vi "zad1.vi"() -> ()   [LabVIEW 2018]
uses:
  Control 6.ctl
  Control 1.ctl
  Control 3.ctl
  <vilib>/measure/maspectr.llb/FFT Power Spectrum and PSD for 1 Chan.vi
  <vilib>/measure/NI_MAPro.lvlib
panel:
  out "Waveform Graph 2":cluster{"f0":dbl, "df":dbl, "magnitude":dbl[]}(graph)
  in  "millisec to wait":u32
  in  "idev 2":u32
  in  "Buffer":T1
  in  "Format":cluster{"Rate":i32, "Bits":i32, "Channels":u32}
  in  "Play":bool
  in  "Exit":bool
  out "Waveform Graph":i32[][](graph)
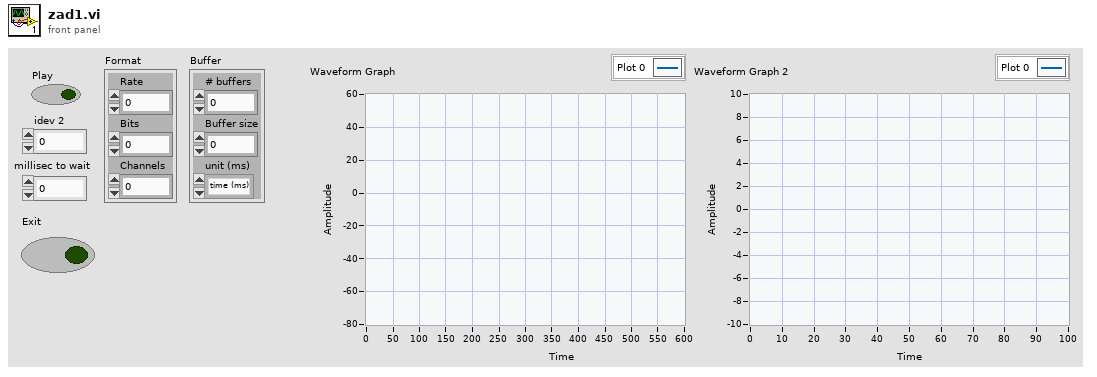
[diagram p1: front panel]
types:
  T1 = cluster{"# buffers":i32, "Buffer size":i32, "unit (ms)":enum16{"time (ms)", "Samples"}}
  T2 = typedef "Control 1.ctl" = enum16{"Analysis", "Initialization", "Idle"}
  T3 = typedef "Control 6.ctl" = enum16{"Idle", "Initialization", "Acquisition", "End"}
  T4 = typedef "Control 3.ctl" = cluster{"Play":bool, "Format (44kHz, 16Bit, stereo)":cluster{"Rate":i32, "Bits":i32, "Channels":u32}, "Buffer Config":cluster{"# buffers":i32, "Buffer size":i32, "unit (ms)":enum16{"time (ms)", "Samples"}}, "idev":u32, "millisec to wait":u32}
  T5 = enum16{"Idle", "Initialization", "Acquisition", "End"}
  T6 = typedef "Control 4.ctl" = cluster{"Play":bool, "Format (44kHz, 16Bit, stereo)":cluster{"Rate":i32, "Bits":i32, "Channels":u32}, "Buffer Config":cluster{"# buffers":i32, "Buffer size":i32, "unit (ms)":enum16{"time (ms)", "Samples"}}, "idev":u32, "millisec to wait":u32}
  T7 = typedef "SoundHandle.ctl" = cluster{"DeviceID":u16, "Samples/buf":u32, "Sampl rate":u32, "Bits/sample":u16, "Channels":u8, "Opened":bool}
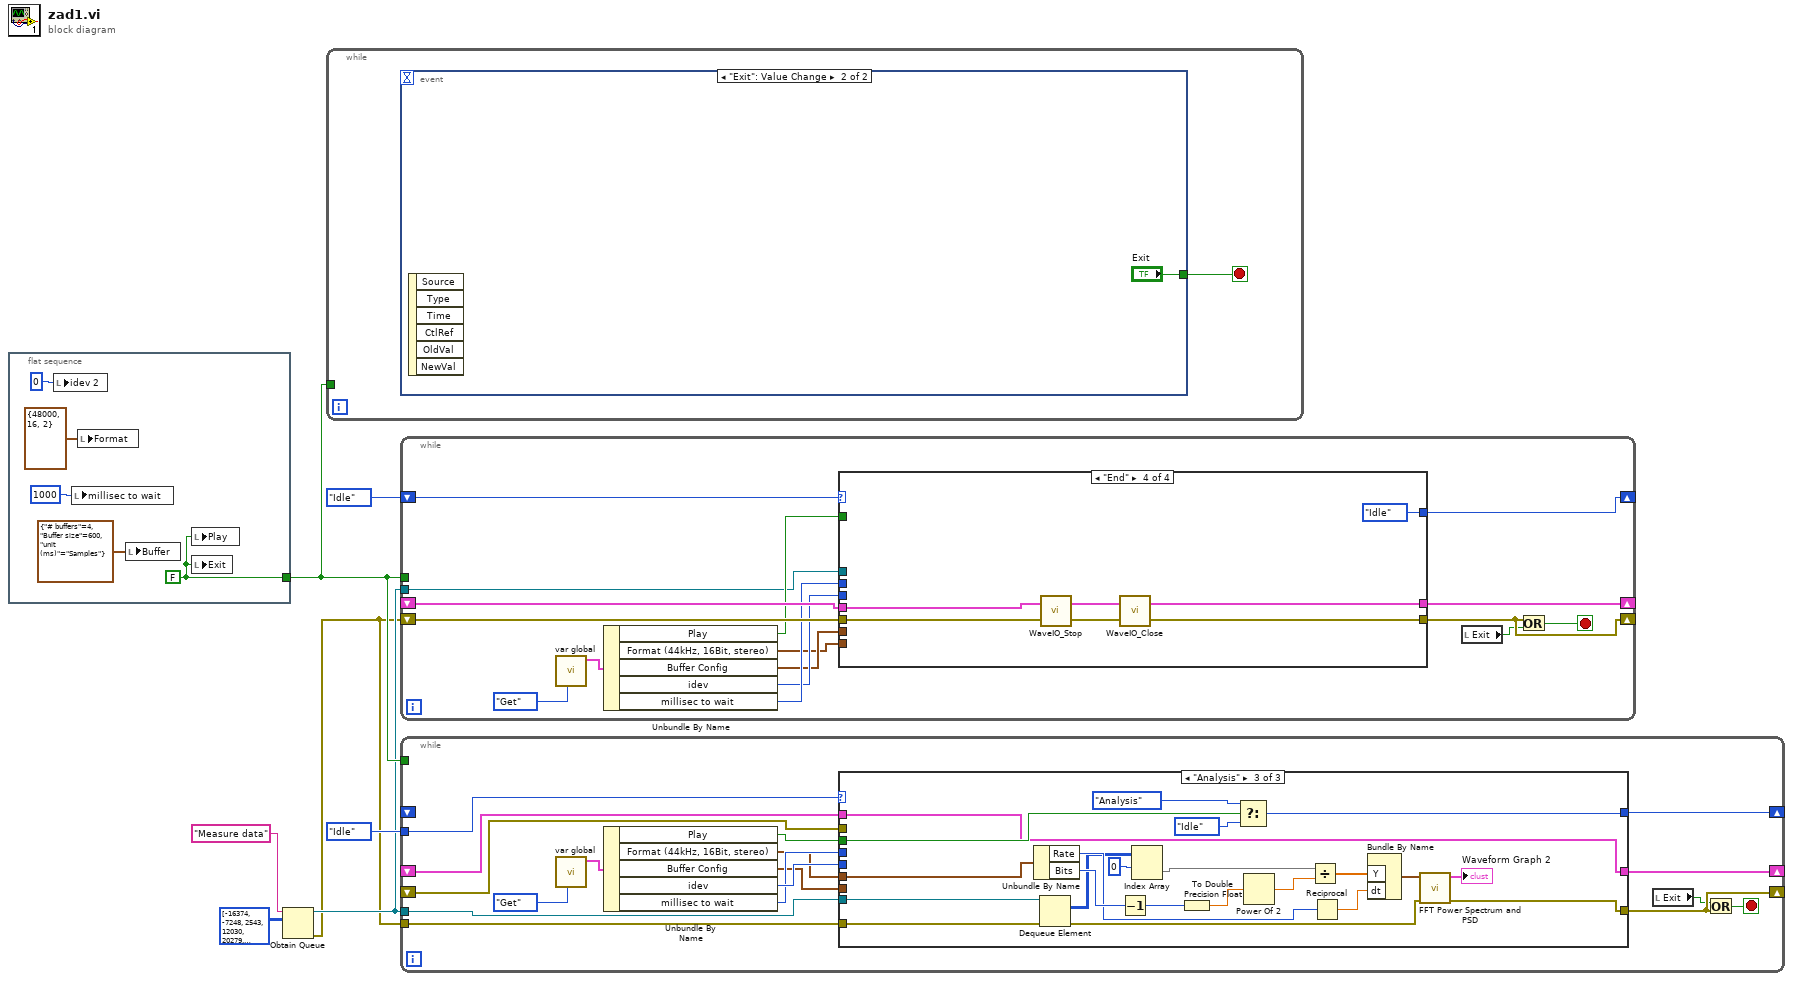
[diagram p0: block diagram]
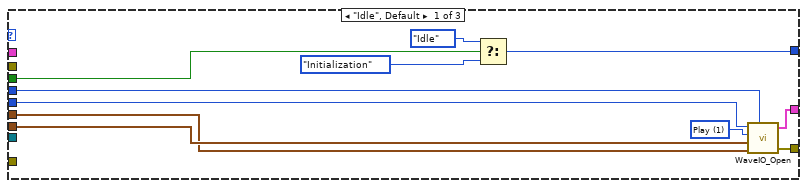
[diagram p2: hidden frame]
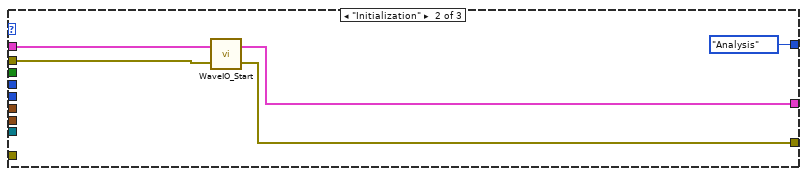
[diagram p3: hidden frame]
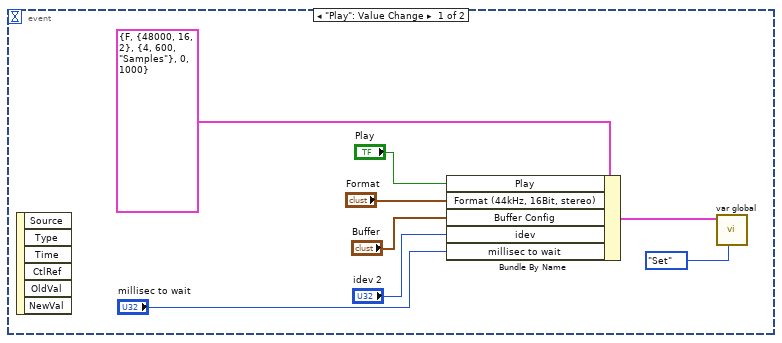
[diagram p4: hidden frame]
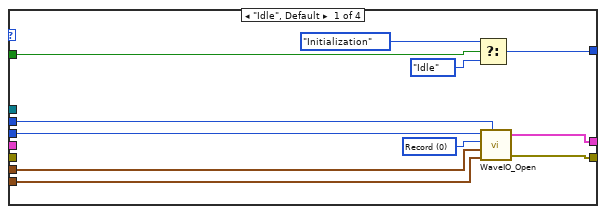
[diagram p5: hidden frame]
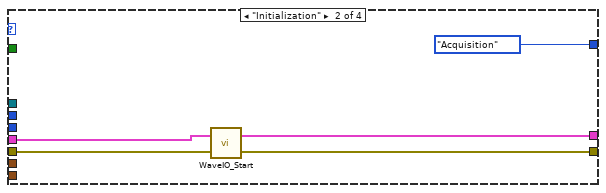
[diagram p6: hidden frame]
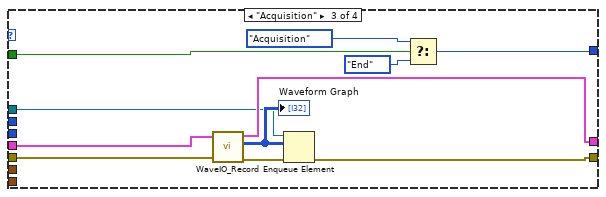
[diagram p7: hidden frame]
diagram:
  n1 = flat-sequence {
    tunnel: [w8] -> w4
    frame #0 {
      w8 = FALSE ("Play")
      n2 = local write "idev 2"(u32 0 ("idev 2")) -> ()
      n3 = local write "millisec to wait"(u32 1000 ("millisec to wait")) -> ()
      n4 = local write "Format"(cluster{"Rate":i32, "Bits":i32, "Channels":u32} {"Rate"=48000, "Bits"=16, "Channels"=2} ("Format")) -> ()
      n5 = local write "Buffer"(T1 {"# buffers"=4, "Buffer size"=600, "unit (ms)"=enum."Samples"} ("Buffer")) -> ()
      n6 = local write "Play"(w8) -> ()
      n7 = local write "Exit"(w8) -> ()
    }
  }
  n8 = Obtain Queue(name (unnamed)="Measure data", element data type=i32[][] [[-16374, -7248, 2543, 12030, 20279, 26487, 30037, 30583, 28073, 22744, 15131, 5976, -3818, -13288, -21504, -27663, -31155, -31636, -29064, -23686, -16036, -6862, 2936, 12388, 20571, 26684, 30122, 30546, 27911, 22483, 14793, 5595, -4207, -13644, -21795, -27855, -31232, -31591, -28898, -23423, -15695, -6476, 3323, 12743, 20858, 26873, 30194, 30492, 27744, 22213, 14447, 5207, -4597, -14002, -22082, -28044, -31304, -31540, -28731, -23149, -15348, -6093, 3713, 13101, 21145, 27063, 30265, 30442, 27576, 21943, 14103, 4822, -4984, -14354, -22365, -28230, -31373, -31485, -28556, -22876, -14998, -5702, 4104, 13452, 21428, 27245, 30335, 30388, 27400, 21669, 13754, 4435, -5375, -14705, -22643, -28407, -31436, -31426, -28378, -22598, -14648, -5314, 4497, 13803, 21706, 27423, 30394, 30325, 27221, 21390, 13402, 4045, -5763, -15056, -22921, -28586, -31496, -31361, -28198, -22319, -14297, -4924, 4879, 14151, 21982, 27597, 30451, 30257, 27038, 21107, 13050, 3658, -6149, -15402, -23193, -28754, -31546, -31290, -28010, -22033, -13944, -4536, 5266, 14498, 22252, 27767, 30500, 30184, 26849, 20821, 12696, 3267, -6535, -15748, -23462, -28924, -31596, -31216, -27821, -21748, -13587, -4147, 5653, 14838, 22519, 27930, 30549, 30110, 26658, 20535, 12337, 2878, -6919, -16089, -23727, -29087, -31641, -31137, -27627, -21457, -13229, -3753, 6038, 15181, 22786, 28093, 30591, 30031, 26461, 20243, 11979, 2485, -7303, -16428, -23991, -29244, -31678, -31053, -27426, -21159, -12867, -3360, 6424, 15524, 23043, 28252, 30633, 29946, 26262, 19946, 11617, 2096, -7686, -16764, -24246, -29398, -31712, -30964, -27224, -20862, -12503, -2971, 6803, 15859, 23301, 28401, 30661, 29852, 26058, 19648, 11254, 1703, -8069, -17099, -24500, -29547, -31741, -30870, -27018, -20562, -12138, -2575, 7188, 16192, 23556, 28549, 30689, 29756, 25848, 19348, 10891, 1312, -8448, -17430, -24753, -29691, -31765, -30773, -26806, -20259, -11775, -2186, 7566, 16521, 23801, 28690, 30709, 29656, 25634, 19038, 10523, 919, -8831, -17762, -24997, -29833, -31788, -30672, -26593, -19955, -11409, -1792, 7944, 16850, 24047, 28830, 30724, 29548, 25416, 18729, 10152, 523, -9212, -18092, -25245, -29969, -31805, -30566, -26375, -19647, -11041, -1403, 8319, 17173, 24287, 28963, 30734, 29436, 25192, 18418, 9781, 130, -9587, -18413, -25481, -30101, -31814, -30449, -26150, -19332, -10666, -1007, 8697, 17497, 24524, 29090, 30745, 29325, 24968, 18105, 9408, -263, -9962, -18735, -25718, -30228, -31820, -30334, -25921, -19016, -10296, -618, 9072, 17814, 24756, 29213, 30746, 29202, 24738, 17787, 9036, -657, -10338, -19058, -25951, -30350, -31818, -30214, -25690, -18699, -9922, -224, 9442, 18128, 24984, 29330, 30738, 29078, 24502, 17466, 8658, -1050, -10710, -19371, -26178, -30467, -31814, -30088, -25458, -18382, -9550, 167, 9812, 18440, 25206, 29443, 30732, 28947, 24264, 17143, 8281, -1445, -11083, -19685, -26404, -30581, -31807, -29959, -25221, -18059, -9175, 556, 10178, 18750, 25426, 29548, 30718, 28809, 24018, 16812, 7901, -1842, -11457, -19996, -26624, -30690, -31795, -29824, -24980, -17733, -8799, 950, 10549, 19058, 25643, 29655, 30700, 28673, 23773, 16484, 7523, -2235, -11824, -20304, -26840, -30793, -31772, -29682, -24731, -17402, -8415, 1341, 10916, 19363, 25856, 29755, 30677, 28528, 23522, 16151, 7141, -2626, -12191, -20607, -27051, -30891, -31746, -29536, -24481, -17070, -8035, 1733, 11280, 19664, 26064, 29851, 30648, 28381, 23272, 15818, 6762, -3019, -12555, -20906, -27258, -30984, -31717, -29391, -24226, -16736, -7655, 2128, 11641, 19962, 26270, 29940, 30615, 28229, 23013, 15483, 6376, -3409, -12914, -21204, -27459, -31071, -31684, -29236, -23967, -16398, -7271, 2515, 12005, 20258, 26468, 30024, 30577, 28072, 22753, 15143, 5990, -3802, -13276, -21497, -27660, -31157, -31643, -29076, -23707, -16058, -6886, 2908, 12363, 20550, 26666, 30107, 30536, 27914, 22489, 14805, 5607, -4192, -13633, -21787, -27849, -31230, -31597, -28911, -23438, -15716, -6501, 3298, 12719, 20839, 26858, 30182, 30488, 27744, 22223, 14459, 5225, -4579, -13988, -22071, -28040, -31304, -31549, -28743, -23167, -15368, -6113, 3693, 13076, 21126, 27047, 30255, 30438, 27576, 21950, 14113, 4837, -4971, -14340, -22354, -28224, -31375, -31494, -28570, -22895, -15022, -5725, 4080, 13430, 21408, 27230, 30324, 30384, 27402, 21676, 13766, 4449, -5360, -14694, -22636, -28409, -31440, -31436, -28397, -22617, -14674, -5338, 4467, 13781, 21686, 27408, 30385, 30320, 27224, 21398, 13418, 4062, -5748, -15044, -22913, -28584, -31498, -31368, -28212, -22339, -14321, -4948, 4856, 14131, 21963, 27583, 30440, 30254, 27042, 21118, 13062, 3669, -6137, -15390, -23183, -28751, -31551, -31297, -28024, -22049, -13962, -4556, 5245, 14476, 22235, 27754, 30497, 30186, 26857, 20834, 12710, 3283, -6519, -15733, -23453, -28921, -31600, -31226, -27837, -21765, -13610, -4168, 5628, 14820, 22502, 27918, 30540, 30109, 26664, 20544, 12354, 2891, -6906, -16074, -23719, -29085, -31646, -31148, -27642, -21475, -13251, -3777, 6014, 15160, 22765, 28078, 30583, 30027, 26468, 20251, 11994, 2501, -7292, -16415, -23980, -29242, -31682, -31064, -27443, -21181, -12892, -3386, 6397, 15501, 23026, 28238, 30624, 29944, 26269, 19959, 11633, 2110, -7673, -16753, -24239, -29395, -31719, -30974, -27239, -20882, -12528, -2993, 6782, 15835, 23285, 28390, 30651, 29852, 26063, 19660, 11271, 1720, -8053, -17087, -24493, -29546, -31746, -30880, -27031, -20583, -12163, -2599, 7166, 16173, 23538, 28538, 30684, 29758, 25853, 19356, 10906, 1327, -8433, -17416, -24743, -29688, -31769, -30782, -26821, -20280, -11797, -2208, 7543, 16501, 23786, 28680, 30704, 29656, 25642, 19053, 10540, 936, -8814, -17747, -24989, -29827, -31787, -30678, -26606, -19973, -11430, -1817, 7923, 16829, 24031, 28819, 30721, 29552, 25424, 18746, 10174, 543, -9191, -18072, -25231, -29962, -31802, -30567, -26384, -19660, -11057, -1422, 8302, 17159, 24274, 28952, 30738, 29443, 25205, 18435, 9801, 150, -9568, -18401, -25472, -30095, -31811, -30457, -26163, -19349, -10687, -1031, 8679, 17481, 24511, 29082, 30742, 29327, 24979, 18121, 9431, -241, -9943, -18717, -25707, -30221, -31815, -30337, -25930, -19029, -10312, -631, 9058, 17802, 24745, 29207, 30746, 29209, 24750, 17805, 9057, -634, -10316, -19037, -25937, -30340, -31814, -30217, -25700, -18713, -9939, -240, 9429, 18117, 24976, 29328, 30740, 29088, 24519, 17486, 8682, -1027, -10688, -19352, -26164, -30458, -31810, -30091, -25465, -18390, -9561, 154, 9800, 18433, 25201, 29442, 30735, 28959, 24282, 17165, 8308, -1420, -11063, -19665, -26386, -30570, -31801, -29961, -25227, -18068, -9185, 547, 10171, 18745, 25424, 29552, 30726, 28825, 24038, 16835, 7925, -1815, -11429, -19974, -26608, -30681, -31789, -29826, -24984, -17741, -8807, 938, 10536, 19047, 25636, 29657, 30708, 28685, 23794, 16510, 7550, -2205, -11798, -20280, -26821, -30782, -31766, -29684, -24737, -17411, -8429, 1331, 10906, 19356, 25851, 29758, 30684, 28544, 23546, 16178, 7169, -2598, -12162, -20582, -27035, -30879, -31744, -29540, -24485, -17080, -8048, 1721, 11267, 19655, 26061, 29852, 30654, 28395, 23291, 15843, 6786, -2993, -12527, -20884, -27240, -30974, -31713, -29390, -24230, -16744, -7662, 2115, 11635, 19957, 26268, 29945, 30624, 28246, 23035, 15509, 6406, -3382, -12889, -21180, -27444, -31061, -31677, -29236, -23975, -16408, -7284], [-19329, -1252, 17344, 29341, 30145, 19451, 1353, -17227, -29174, -29920, -19175, -1056, 17506, 29408, 30095, 19300, 1159, -17387, -29238, -29860, -19019, -860, 17671, 29475, 30037, 19143, 960, -17553, -29307, -29809, -18866, -664, 17832, 29545, 29987, 18991, 771, -17707, -29365, -29749, -18707, -466, 17992, 29605, 29926, 18832, 570, -17873, -29434, -29694, -18556, -272, 18151, 29670, 29869, 18676, 375, -18031, -29495, -29633, -18395, -75, 18310, 29729, 29809, 18516, 175, -18194, -29561, -29579, -18238, 120, 18469, 29792, 29750, 18362, -17, -18347, -29617, -29515, -18076, 316, 18629, 29848, 29682, 18197, -218, -18510, -29679, -29456, -17921, 513, 18787, 29910, 29626, 18042, -408, -18664, -29734, -29388, -17757, 709, 18941, 29965, 29560, 17875, -609, -18823, -29791, -29326, -17600, 904, 19095, 30023, 29495, 17717, -802, -18975, -29845, -29260, -17434, 1099, 19251, 30075, 29425, 17551, -1001, -19131, -29901, -29194, -17277, 1296, 19408, 30130, 29359, 17393, -1193, -19284, -29953, -29124, -17112, 1491, 19560, 30184, 29290, 17225, -1392, -19440, -30008, -29056, -16949, 1686, 19713, 30237, 29226, 17069, -1581, -19587, -30054, -28982, -16781, 1883, 19866, 30287, 29151, 16898, -1781, -19742, -30107, -28913, -16616, 2079, 20018, 30337, 29082, 16737, -1973, -19888, -30152, -28838, -16449, 2275, 20167, 30383, 29006, 16564, -2174, -20041, -30200, -28765, -16282, 2471, 20321, 30430, 28934, 16403, -2364, -20187, -30243, -28688, -16113, 2669, 20465, 30470, 28853, 16230, -2568, -20341, -30294, -28618, -15953, 2860, 20615, 30519, 28783, 16070, -2755, -20486, -30335, -28537, -15779, 3057, 20760, 30560, 28700, 15892, -2956, -20637, -30378, -28461, -15613, 3252, 20909, 30605, 28628, 15730, -3145, -20777, -30418, -28377, -15440, 3446, 21054, 30645, 28543, 15557, -3345, -20927, -30460, -28299, -15271, 3643, 21199, 30686, 28465, 15391, -3534, -21066, -30495, -28215, -15100, 3839, 21345, 30722, 28380, 15214, -3734, -21213, -30534, -28134, -14928, 4032, 21487, 30760, 28300, 15044, -3926, -21355, -30570, -28052, -14757, 4225, 21627, 30792, 28209, 14870, -4123, -21501, -30607, -27968, -14586, 4419, 21768, 30832, 28129, 14702, -4314, -21637, -30639, -27880, -14413, 4612, 21907, 30859, 28040, 14521, -4515, -21780, -30675, -27796, -14241, 4804, 22048, 30895, 27953, 14352, -4702, -21919, -30705, -27707, -14064, 4999, 22187, 30922, 27859, 14172, -4900, -22060, -30739, -27620, -13892, 5193, 22326, 30954, 27773, 14003, -5090, -22194, -30765, -27524, -13712, 5386, 22462, 30981, 27679, 13823, -5285, -22333, -30794, -27436, -13538, 5580, 22600, 31013, 27591, 13650, -5476, -22466, -30820, -27343, -13363, 5770, 22732, 31033, 27491, 13468, -5673, -22605, -30848, -27251, -13187, 5964, 22870, 31060, 27401, 13292, -5863, -22736, -30870, -27155, -13010, 6156, 23000, 31079, 27299, 13111, -6058, -22873, -30895, -27060, -12833, 6347, 23134, 31104, 27208, 12936, -6248, -23004, -30918, -26965, -12652, 6536, 23260, 31120, 27106, 12753, -6444, -23136, -30939, -26865, -12472, 6729, 23395, 31148, 27011, 12578, -6634, -23266, -30959, -26766, -12296, 6919, 23523, 31161, 26907, 12392, -6830, -23402, -30982, -26665, -12115, 7109, 23652, 31180, 26809, 12213, -7016, -23524, -30992, -26564, -11932, 7301, 23777, 31195, 26704, 12032, -7210, -23655, -31011, -26464, -11755, 7492, 23907, 31211, 26605, 11855, -7395, -23778, -31024, -26358, -11573, 7680, 24031, 31218, 26494, 11665, -7592, -23908, -31039, -26258, -11392, 7871, 24158, 31237, 26394, 11491, -7775, -24031, -31050, -26153, -11210, 8063, 24281, 31247, 26285, 11302, -7972, -24159, -31062, -26046, -11027, 8250, 24407, 31258, 26180, 11124, -8157, -24276, -31067, -25937, -10841, 8438, 24526, 31265, 26071, 10936, -8347, -24401, -31078, -25829, -10659, 8630, 24649, 31275, 25965, 10755, -8533, -24522, -31087, -25721, -10474, 8816, 24770, 31280, 25853, 10566, -8726, -24641, -31091, -25608, -10290, 9003, 24891, 31287, 25746, 10386, -8910, -24756, -31095, -25498, -10105, 9192, 25008, 31287, 25627, 10196, -9102, -24881, -31101, -25386, -9919, 9381, 25127, 31296, 25521, 10019, -9284, -24994, -31099, -25268, -9732, 9570, 25243, 31293, 25403, 9826, -9476, -25113, -31105, -25157, -9544, 9756, 25359, 31298, 25291, 9645, -9655, -25225, -31099, -25040, -9359, 9942, 25473, 31291, 25167, 9453, -9847, -25341, -31102, -24926, -9173, 10124, 25586, 31294, 25057, 9269, -10029, -25450, -31095, -24809, -8986, 10310, 25696, 31284, 24931, 9078, -10218, -25564, -31094, -24688, -8798, 10497, 25812, 31287, 24819, 8896, -10399, -25673, -31085, -24567, -8608, 10682, 25922, 31278, 24698, 8703, -10587, -25785, -31080, -24448, -8422, 10866, 26033, 31274, 24582, 8522, -10765, -25890, -31067, -24321, -8230, 11050, 26140, 31263, 24455, 8325, -10952, -26001, -31064, -24201, -8040, 11234, 26248, 31255, 24338, 8142, -11132, -26106, -31054, -24079, -7852, 11417, 26353, 31243, 24207, 7948, -11316, -26217, -31041, -23952, -7662, 11601, 26464, 31236, 24089, 7763, -11494, -26315, -31025, -23829, -7471, 11782, 26562, 31217, 23957, 7567, -11682, -26422, -31014, -23702, -7282, 11962, 26667, 31205, 23834, 7383, -11859, -26521, -30998, -23575, -7092, 12144, 26770, 31187, 23704, 7186, -12043, -26626, -30981, -23444, -6900, 12328, 26875, 31176, 23582, 7003, -12218, -26724, -30962, -23316, -6709, 12505, 26971, 31154, 23446, 6805, -12401, -26825, -30946, -23189, -6517, 12687, 27073, 31139, 23322, 6620, -12576, -26919, -30922, -23054, -6323, 12867, 27170, 31114, 23185, 6422, -12760, -27022, -30904, -22923, -6132, 13047, 27272, 31096, 23060, 6237, -12934, -27114, -30879, -22790, -5940, 13222, 27362, 31068, 22921, 6041, -13116, -27212, -30855, -22657, -5748, 13401, 27461, 31048, 22790, 5853, -13289, -27302, -30828, -22522, -5555, 13577, 27549, 31019, 22652, 5652, -13472, -27398, -30806, -22388, -5362, 13753, 27645, 30995, 22521, 5463, -13642, -27487, -30776, -22248, -5169, 13928, 27733, 30963, 22376, 5266, -13823, -27584, -30750, -22113, -4975, 14106, 27828, 30937, 22246, 5082, -13992, -27669, -30717, -21974, -4782, 14280, 27914, 30902, 22101, 4880, -14174, -27760, -30689, -21837, -4588, 14454, 28006, 30875, 21965, 4692, -14340, -27843, -30653, -21693, -4391, 14631, 28092, 30840, 21822, 4494, -14519, -27934, -30620, -21552, -4198, 14805, 28179, 30808, 21688, 4308, -14687, -28015, -30582, -21410, -4004, 14975, 28262, 30770, 21540, 4106, -14861, -28103, -30548, -21268, -3808, 15149, 28349, 30739, 21402, 3916, -15032, -28183, -30512, -21124, -3614, 15319, 28430, 30697, 21255, 3715, -15205, -28267, -30475, -20982, -3421, 15490, 28513, 30664, 21116, 3524, -15376, -28348, -30435, -20837, -3225, 15660, 28592, 30617, 20962, 3327, -15550, -28432, -30397, -20695, -3032, 15829, 28673, 30581, 20820, 3134, -15711, -28506, -30353, -20546, -2837, 15994, 28746, 30530, 20669, 2933, -15887, -28585, -30311, -20400, -2641, 16167, 28828, 30496, 20528, 2745, -16052, -28660, -30264, -20248, -2445, 16335, 28901, 30445, 20376, 2544, -16221, -28737, -30219, -20102, -2250, 16505, 28983, 30406, 20231, 2357, -16381, -28808, -30171, -19950, -2053, 16670, 29053, 30355, 20075, 2154, -16552, -28883, -30127, -19803, -1859, 16835, 29128, 30308, 19930, 1965, -16714, -28952, -30073, -19650, -1663, 17001, 29192, 30255, 19772, 1764, -16881, -29028, -30026, -19496, -1467, 17165, 29268, 30208, 19626, 1572, -17043, -29095, -29977, -19346]] ("Data")) -> (queue out=w2:refnum<queue>, error out=w1:errorcluster)  [unwired: 3 in, 1 out]
  n9 = while {
    tunnel: w4 -> [_]
    stop <- w13 stop-if-true
    n10 = event shown="[1] \"Exit\": Value Change" {
      selector: _ -> [_ _]
      dyn-events: _ -> [_ _]
      timeout: _ -> [_ _]
      tunnel: [_ "Exit"] -> w13
      event "Play": Value Change {
        n11 = event-data() -> ()  [unwired: 1 in, 6 out]
        n12 = Bundle By Name(cluster=T4 {"Play"=FALSE, "Format (44kHz, 16Bit, stereo)"={"Rate"=48000, "Bits"=16, "Channels"=2}, "Buffer Config"={"# buffers"=4, "Buffer size"=600, "unit (ms)"=enum."Samples"}, "idev"=0, "millisec to wait"=1000} ("input"), "Play"="Play", "Format (44kHz, 16Bit, stereo)"="Format", "Buffer Config"="Buffer", "idev"="idev 2", "millisec to wait"="millisec to wait") -> (w14:T4)
        n13 = call "var global.vi"("Action"=enum16{"Set", "Get"}."Set", "input"=w14) -> ()  [unwired: 9 in, 1 out]
      }
      event "Exit": Value Change {
        n14 = event-data() -> ()  [unwired: 1 in, 6 out]
      }
    }
  }
  n15 = while {
    shift-right: [w37] -> _
    shift-left: Control_6."Idle" -> [w38]
    shift-right: [w35] -> _
    shift-left: _ -> [w34]
    shift-right: [w32] -> _
    shift-left: w1 -> [w33]
    tunnel: w4 -> [_]
    tunnel: w2 -> [w24]
    stop <- w36 stop-if-true
    n16 = call "var global.vi"("Action"=enum16{"Set", "Get"}."Get") -> ("output"=w31:T6)  [unwired: 10 in]
    n17 = Unbundle By Name(w31) -> ("Play"=w29:bool, "Format (44kHz, 16Bit, stereo)"=w25:cluster{"Rate":i32, "Bits":i32, "Channels":u32}, "Buffer Config"=w26:T1, "idev"=w27:u32, "millisec to wait"=w28:u32)
    n18 = case shown="\"End\"" w38 {
      tunnel: [w49 T5."Acquisition" w65 T5."Idle"] -> w37
      tunnel: [w47 w51 w60 w66] -> w35
      tunnel: [w46 w50 w56 w67] -> w32
      tunnel: w34 -> [_ w53 w62 w71]
      tunnel: w33 -> [_ w52 w61 w70]
      tunnel: w29 -> [w45 _ w59 _]
      tunnel: w28 -> [w44 _ _ _]
      tunnel: w27 -> [w43 _ _ _]
      tunnel: w26 -> [w42 _ _ _]
      tunnel: w25 -> [w41 _ _ _]
      tunnel: w24 -> [_ _ w55 _]
      frame "Idle", Default {
        w48 = u16 0 items=["Record", "Play", "Loopback", "ASIO input", "ASIO output", "Record (WASAPI)", "Play (WASAPI)", "Record Combi", "Play Combi"] ("device type (Record)")
        n19 = Select(t=T5."Initialization", s=w45, f=T5."Idle") -> (s? t:f=w49:T5)
        n20 = call "WaveIO_Open.vi"("idev"=w43, "Watchdog timeout (msec) (default=OFF)"=w44, "device type (Record)"=w48, "Buffer Config"=w42, "Format (44kHz, 16Bit, stereo)"=w41) -> ("Sound Handle Out"=w47:T7, "error out"=w46:errorcluster)  [unwired: 2 in]
      }
      frame "Initialization" {
        n21 = call "WaveIO_Start.vi"("error in (no error)"=w52, "Handle"=w53) -> ("error out"=w50:errorcluster, "Handle Out"=w51:T7)
      }
      frame "Acquisition" {
        n22 = call "WaveIO_Record.vi"("Handle"=w62, "error in (no error)"=w61) -> ("Handle Out"=w60:T7, "Data"=w58:i32[][], "error out"=w57:errorcluster)  [unwired: 1 in, 2 out]
        "Waveform Graph" <- w58
        n23 = Enqueue Element(queue=w55, element=w58, error in (no error)=w57) -> (error out=w56:errorcluster)  [unwired: 1 in, 2 out]
        n24 = Select(t=T5."Acquisition", s=w59, f=T5."End") -> (s? t:f=w65:T5)
      }
      frame "End" {
        n25 = call "WaveIO_Stop.vi"("error in (no error)"=w70, "Handle"=w71) -> ("error out"=w68:errorcluster, "Handle Out"=w69:T7)
        n26 = call "WaveIO_Close.vi"("error in (no error)"=w68, "Handle"=w69) -> ("error out"=w67:errorcluster, "Handle Out"=w66:T7)
      }
    }
    n27 = local read "Exit"() -> (w23:bool)
    n28 = Or(x=w32, y=w23) -> (x .or. y?=w36:bool)
  }
  n29 = while {
    tunnel: w4 -> [_]
    tunnel: Control_1."Idle" -> [w89]
    shift-right: [w81] -> _
    shift-left: _ -> [_]
    shift-right: [w80] -> _
    shift-left: _ -> [w78]
    shift-right: [w75] -> _
    shift-left: _ -> [w79]
    tunnel: w2 -> [w77]
    tunnel: w1 -> [w76]
    stop <- w73 stop-if-true
    n30 = call "var global.vi"("Action"=enum16{"Set", "Get"}."Get") -> ("output"=w88:T6)  [unwired: 10 in]
    n31 = Unbundle By Name(w88) -> ("Play"=w82:bool, "Format (44kHz, 16Bit, stereo)"=w83:cluster{"Rate":i32, "Bits":i32, "Channels":u32}, "Buffer Config"=w84:T1, "idev"=w86:u32, "millisec to wait"=w85:u32)
    n32 = case shown="\"Analysis\"" w89 {
      tunnel: w86 -> [w100 _ _]
      tunnel: w85 -> [w90 _ _]
      tunnel: w84 -> [w99 _ _]
      tunnel: w83 -> [w98 _ w123]
      tunnel: w82 -> [w96 _ w124]
      tunnel: [w94 enum16{"Analysis", "Initialization", "Idle"}."Analysis" w127] -> w81
      tunnel: [w93 w102 w111] -> w80
      tunnel: [w92 w104 w110] -> w75
      tunnel: w79 -> [_ w105 _]
      tunnel: w78 -> [_ w103 w111]
      tunnel: w77 -> [_ _ w116]
      tunnel: w76 -> [_ _ w115]
      frame "Idle", Default {
        w91 = u16 1 items=["Record", "Play", "Loopback", "ASIO input", "ASIO output", "Record (WASAPI)", "Play (WASAPI)", "Record Combi", "Play Combi"] ("device type (Record)")
        n33 = Select(t=T5."Idle", s=w96, f=enum16{"Analysis", "Initialization", "Idle"}."Initialization") -> (s? t:f=w94:u16)
        n34 = call "WaveIO_Open.vi"("idev"=w100, "Watchdog timeout (msec) (default=OFF)"=w90, "device type (Record)"=w91, "Buffer Config"=w99, "Format (44kHz, 16Bit, stereo)"=w98) -> ("Sound Handle Out"=w93:T7, "error out"=w92:errorcluster)  [unwired: 2 in]
      }
      frame "Initialization" {
        n35 = call "WaveIO_Start.vi"("error in (no error)"=w105, "Handle"=w103) -> ("error out"=w104:errorcluster, "Handle Out"=w102:T7)
      }
      frame "Analysis" {
        n36 = Unbundle By Name(w123) -> ("Rate"=w119:i32, "Bits"=w122:i32)
        n37 = Dequeue Element(queue=w116, error in (no error)=w115) -> (element=w113:i32[][], error out=w109:errorcluster)  [unwired: 1 in, 2 out]
        n38 = Decrement(x=w122) -> (x-1=w121:i32)
        n39 = Index Array(array=w113, index (row)=0 ("index")) -> (element=w106:i32[])  [unwired: 1 in]
        n40 = To Double Precision Float(number=w121) -> (double precision float=w120:dbl)
        n41 = Select(t=enum16{"Analysis", "Initialization", "Idle"}."Analysis", s=w124, f=enum16{"Analysis", "Initialization", "Idle"}."Idle") -> (s? t:f=w127:enum16{"Analysis", "Initialization", "Idle"})
        n42 = Power Of 2(x=w120) -> (2^x=w117:dbl)
        n43 = Divide(x=w106, y=w117) -> (x/y=w114:dbl[])
        n44 = Reciprocal(x=w119) -> (1/x=w118:dbl)
        n45 = Bundle By Name("Y"=w114, "dt"=w118) -> (w108:waveform(dbl))  [unwired: 1 in]
        n46 = call-poly <vilib>:"FFT Power Spectrum and PSD.vi"("error in (no error)"=w109, "time signal"=w108) -> ("error out"=w110:errorcluster, "Power Spectrum / PSD"=→"Waveform Graph 2":cluster{"f0":dbl, "df":dbl, "magnitude":dbl[]})  [unwired: 6 in, 2 out]
      }
    }
    n47 = local read "Exit"() -> (w74:bool)
    n48 = Or(x=w74, y=w75) -> (x .or. y?=w73:bool)
  }
